vi "5.10 Improved Covariance.vi"(2 "Scaling":dbl[](array[numeric]), 3 "X":dbl[][](array[numeric])) -> (0 "mean vector":dbl[](array[numeric]), 1 "covariance matrix V":T1)   [LabVIEW 2011]
uses:
  <vilib>/Analysis/Matrix/Datatypes/RealMatrix.ctl
  <vilib>/Analysis/Matrix/Numeric/Multiply/Multiply - RM,R.vi
  <vilib>/Analysis/baseanly.llb/Real Outer Product.vi
  <vilib>/Analysis/Matrix/Numeric/Multiply/Multiply - R,RM.vi
  <vilib>/Analysis/Matrix/Numeric/Add/Add - RM,RM.vi
  <vilib>/Analysis/NI_AALBase.lvlib
  <vilib>/Analysis/Matrix/NI_Matrix.lvlib
panel:
  out "1/x":dbl
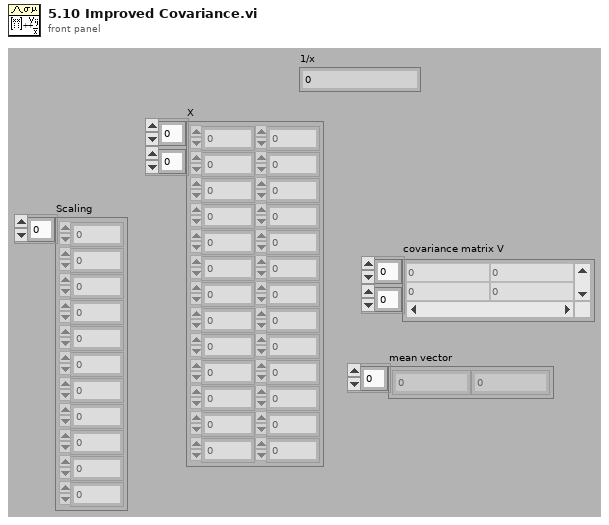
[diagram p1: front panel]
types:
  T1 = typedef "NI_Matrix.lvlib/RealMatrix.ctl" = dbl[][]
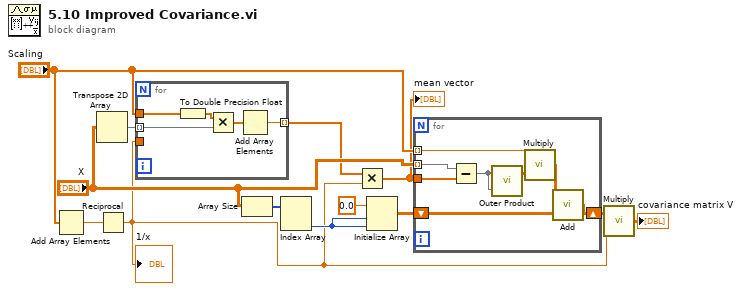
[diagram p0: block diagram]
diagram:
  n1 = Add Array Elements(numeric array="Scaling") -> (sum=w1:dbl)
  n2 = Transpose 2D Array(2D array="X") -> (transposed array=w8:dbl[][])
  n3 = Reciprocal(x=w1) -> (1/x=w2:dbl)
  "1/x" <- w2
  n4 = for {
    tunnel: w8 -> [w18] mode=indexing
    tunnel: [w14] -> w4 mode=indexing
    tunnel: "Scaling" -> [w16]
    tunnel: w2 -> [_]
    n5 = To Double Precision Float(number=w16) -> (double precision float=w15:dbl[])
    n6 = Multiply(x=w15, y=w18) -> (x*y=w17:dbl[])
    n7 = Add Array Elements(numeric array=w17) -> (sum=w14:dbl)
  }
  n8 = Array Size(array="X") -> (size(s)=w11:i32[])
  n9 = Index Array(array=w11) -> (element #2=w9:i32)  [unwired: 2 in, 1 out]
  n10 = Multiply(x=w4, y=w2) -> (x*y=w3:dbl[])
  "mean vector" <- w3
  n11 = Initialize Array(0.0 ("element"), w9, w9) -> (w13:dbl[][])
  n12 = for {
    tunnel: "X" -> [w25] mode=indexing
    tunnel: w3 -> [w26]
    shift-right: [w22] -> w6
    shift-left: w13 -> [w23]
    tunnel: "Scaling" -> [w19] mode=indexing
    n13 = Subtract(x=w25, y=w26) -> (x-y=w21:dbl[])
    n14 = call-poly <vilib>:"Outer Product.vi"("Y Vector"=w21, "X Vector"=w21) -> ("Outer Product"=w24:T1)  [unwired: 1 out]
    n15 = call-poly <vilib>:"Multiply.vi"("Real Matrix A"=w24, "Real Scalar c"=w19) -> ("c * A"=w20:T1)
    n16 = call-poly <vilib>:"Add.vi"("Real Matrix B"=w23, "Real Matrix A"=w20) -> ("A + B"=w22:T1)
  }
  n17 = call-poly <vilib>:"Multiply.vi"("Real Scalar c"=w2, "Real Matrix A"=w6) -> ("A * c"=→"covariance matrix V":T1)
